vi "InitializeRebootLog.vi"(8 "error in (no error)":errorcluster) -> (0 "error out":errorcluster, 2 "log string":string="Reboot count exceeds limit, setting safe mode", 3 "reboot count limit met":bool)   [LabVIEW 2017, in "Controller.lvlib"]
uses:
  <vilib>/addons/InsightCM/Devices/Shared/Common/Controller/Controller.lvlib
  <vilib>/addons/InsightCM/Devices/Shared/Common/Controller/controls/operations.ctl
  <vilib>/addons/InsightCM/Utilities/GlobalConfiguration/GlobalConfiguration.lvlib
  <vilib>/addons/InsightCM/Utilities/PropertyHelpers/PropertyHelpers.lvlib
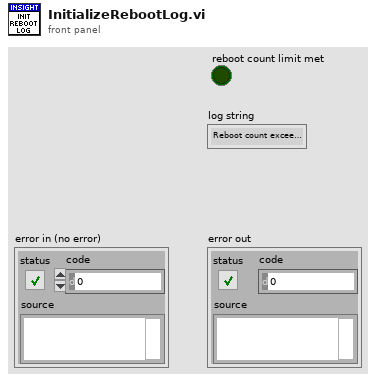
[diagram p1: front panel]
types:
  T1 = typedef "Controller.lvlib/operations.ctl" = enum16{"Unknown", "Startup", "Expected Shutdown"}
  T2 = typedef "SectionKeyValues.ctl" = cluster{"Section":string, "KeyValues":T3[]}
  T3 = typedef "KeyValuePair.ctl" = cluster{"Key":string, "Value":string}
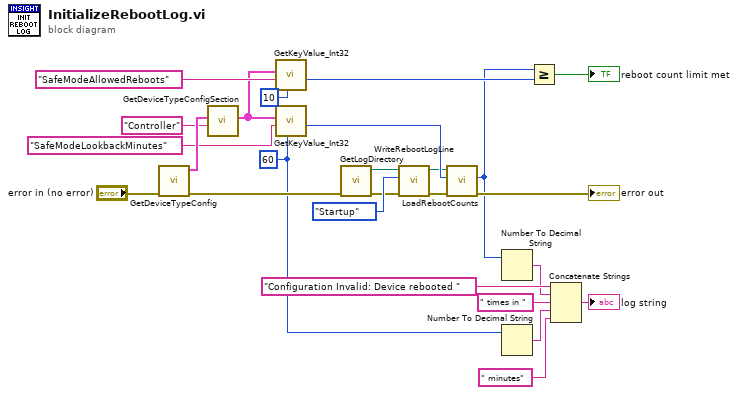
[diagram p0: block diagram]
diagram:
  w8 = 60 ("default")
  n1 = call <vilib>:"GetDeviceTypeConfig.vi"("error in (no error)"="error in (no error)") -> ("error out"=w23:errorcluster, "key values"=w22:T2[])  [unwired: 8 in, 1 out]
  n2 = call <vilib>:"GetDeviceTypeConfigSection.vi"("key"="Controller", "key values"=w22) -> ("key value pairs out"=w17:T3[])  [unwired: 8 in, 1 out]
  n3 = call <vilib>:"GetKeyValue_Int32.vi"("default"=10, "key"="SafeModeAllowedReboots", "key value pairs"=w17) -> ("value"=w18:i32)  [unwired: 6 in, 2 out]
  n4 = call <vilib>:"GetKeyValue_Int32.vi"("default"=w8, "key"="SafeModeLookbackMinutes", "key value pairs"=w17) -> ("value"=w14:i32)  [unwired: 6 in, 2 out]
  n5 = call <vilib>:"GetLogDirectory.vi"("error in (no error)"=w23) -> ("error out"=w6:errorcluster, "log dir"=w4:path)  [unwired: 9 in]
  n6 = call <vilib>:"WriteRebootLogLine.vi"("error in"=w6, "operation"=operations."Startup", "log path"=w4) -> ("error out"=w5:errorcluster, "log path out"=w3:path)  [unwired: 7 in]
  n7 = call <vilib>:"LoadRebootCounts.vi"("error in (no error)"=w5, "lookback minutes"=w14, "log dir"=w3) -> ("error out"=→"error out":errorcluster, "reboot count"=w1:i32)  [unwired: 6 in, 1 out]
  n8 = Number To Decimal String(number=w1) -> (decimal integer string=w13:string)  [unwired: 1 in]
  n9 = Number To Decimal String(number=w8) -> (decimal integer string=w10:string)  [unwired: 1 in]
  n10 = Greater Or Equal?(x=w1, y=w18) -> (x >= y?=→"reboot count limit met":bool)
  n11 = Concatenate Strings("Configuration Invalid: Device rebooted " ("log string"), w13, " times in " ("string"), w10, " minutes" ("string")) -> (→"log string":string)
